vi "S2DS_Select Instrument to edit (SubVI).vi"(8 "error in (no error)":errorcluster, 10 "Available edit instruments":string[](array[string])) -> (0 "error out":errorcluster, 2 "Discard?":bool, 3 "Selected instrument":string)   [LabVIEW 2025]
panel:
  in  "Select instrument":string(combo)
  in  "stop":bool
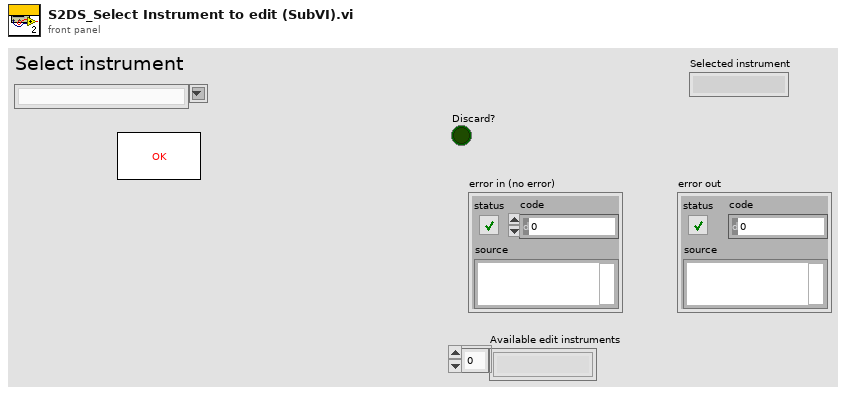
[diagram p1: front panel]
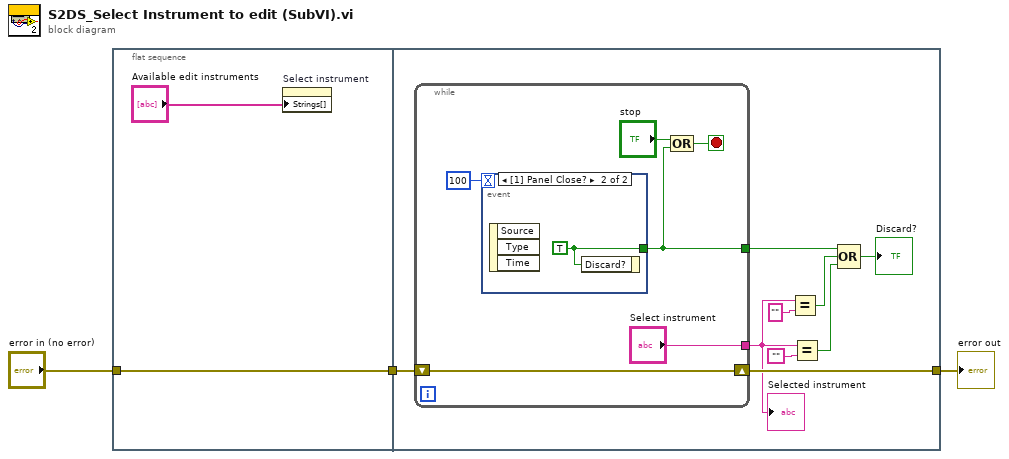
[diagram p0: block diagram]
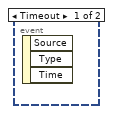
[diagram p2: hidden frame]
diagram:
  n1 = flat-sequence {
    tunnel: [w5] -> w3
    tunnel: "error in (no error)" -> [w5]
    tunnel: w3 -> [w14]
    tunnel: [w13] -> w1
    frame #0 {
      n2 = property on="Select instrument" class="CmbBox"("Strings[]"="Available edit instruments") -> ()  [unwired: 2 in, 2 out]
    }
    frame #1 {
      n3 = while {
        tunnel: [w17] -> w9
        tunnel: ["Select instrument"] -> w11
        shift-right: [w15] -> w13
        shift-left: w14 -> [w15]
        stop <- w18 stop-if-true
        n4 = event shown="[1] Panel Close?" {
          selector: _ -> [_ _]
          dyn-events: _ -> [_ _]
          timeout: 100 -> [_ _]
          tunnel: [_ w21] -> w17
          event Timeout {
            n5 = event-data() -> ()  [unwired: 1 in, 3 out]
          }
          event Panel Close? {
            w21 = TRUE ("Discard?")
            n6 = event-data() -> ()  [unwired: 1 in, 3 out]
            n7 = event-data("Discard?"=w21) -> ()  [unwired: 1 in, 1 out]
          }
        }
        n8 = Compound Arithmetic op=OR("stop", w17) -> (w18:bool)
      }
      "Selected instrument" <- w11
      n9 = Equal?(x=w11, y="") -> (x = y?=w8:bool)
      n10 = Equal?(x=w11, y="") -> (x = y?=w7:bool)
      n11 = Compound Arithmetic op=OR(w9, w8, w7) -> (→"Discard?":bool)
    }
  }
  "error out" <- w1
